vi "play_Sound.vi"(0 "Schrittweite [µm]":u16) -> ()   [LabVIEW 2009]
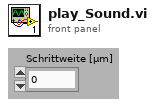
[diagram p1: front panel]
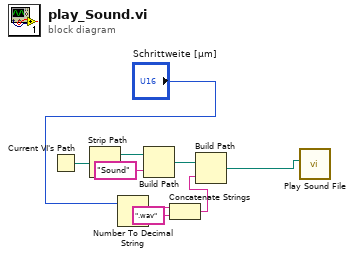
[diagram p0: block diagram]
diagram:
  n1 = Current VI's Path() -> (path=w1:path)
  n2 = Strip Path(path=w1) -> (stripped path=w2:path)  [unwired: 1 out]
  n3 = Number To Decimal String(number="Schrittweite [µm]") -> (decimal integer string=w5:string)  [unwired: 1 in]
  n4 = Build Path(base path=w2, name or relative path="Sound" ("Name oder relativer Pfad")) -> (appended path=w4:path)
  n5 = Concatenate Strings(w5, ".wav" ("String")) -> (w7:string)
  n6 = Build Path(base path=w4, name or relative path=w7) -> (appended path=w8:path)
  n7 = call <vilib>:"Play Sound File.vi"("path"=w8) -> ()  [unwired: 9 in, 2 out]
